vi "Multify(SGL).vi"(1 "启用（T）":bool=TRUE, 2 "In":sgl, 4 "n":sgl=1.0) -> (6 "Out":sgl=1.0 format="%.2f")   [LabVIEW 2011]
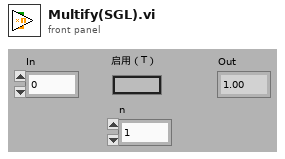
[diagram p1: front panel]
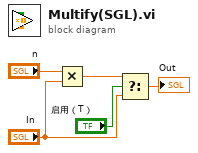
[diagram p0: block diagram]
diagram:
  n1 = Multiply(x="n", y="In") -> (x*y=w1:sgl)
  n2 = Select(t=w1, s="启用（T）", f="In") -> (s? t:f=→"Out":sgl)
